vi "AO 1 Samples FPGA（Host）.vi"() -> ()   [LabVIEW 2019]
uses:
  <vilib>/FPGAPlugInAG/ELVIS III/niLvFpga_Open_ELVIS III.vi
  <vilib>/rvi/interface/common/dynamic/niFpgaDynamicAddResources.vi
  <vilib>/Utility/error.llb/Error Cluster From Error Code.vi
  <vilib>/rvi/errors/niLvFpgaAdjustHostInterfaceError.vi
  <vilib>/FPGAPlugInAG/Dynamic/niLvFpga_Run_Dynamic.vi
  <vilib>/FPGAPlugInAG/Dynamic/niLvFpga_Close_Dynamic.vi
  <vilib>/rvi/interface/nirviOpenFPGA/nirviOpenFPGA.xnode
  FPGA Bitfiles/analogio-fpga_FPGATarget_AO1SamplesFPGA_Fh4Y4n0B4rI.lvbitx
  AO 1 Samples FPGA.vi
  <vilib>/rvi/interface/nirviReadWriteControl/nirviReadWriteControl.xnode
  <vilib>/rvi/interface/nirviMethod/nirviMethod.xnode
  <vilib>/rvi/interface/nirviCloseFPGA/nirviCloseFPGA.xnode
  NiFpgaLv.dll
  <vilib>/rvi/interface/Simulation/niFpgaSimulationCallBeginRW.vi
panel:
  in  "停止":bool
  in  "B1":dbl
  in  "B0":dbl
  in  "A1":dbl
  in  "A0":dbl
  in  "Enable":bool[](array[boolean])=[TRUE, FALSE, FALSE, FALSE]
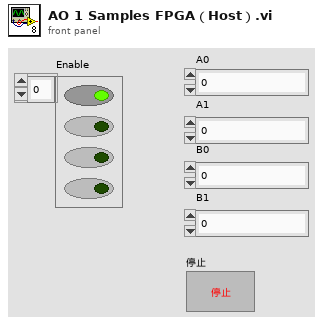
[diagram p1: front panel]
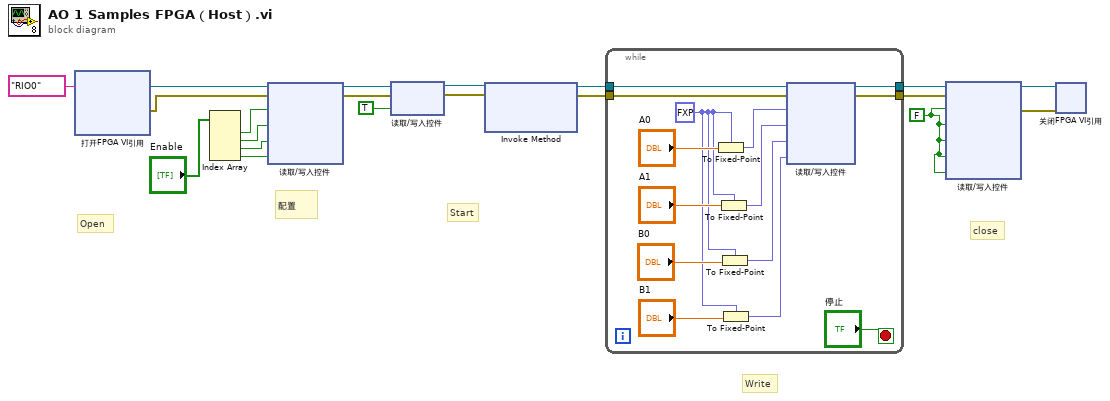
[diagram p0: block diagram]
diagram:
  w1 = FALSE
  # "Open"
  # "close"
  # "Write"
  # "Start"
  # "配置"
  n1 = xnode "打开FPGA VI引用"("资源名称"=tag "RIO0") -> ("FPGA VI引用输出"=w18:refnum<k20>, "错误输出"=w17:errorcluster)  [unwired: 1 in]
  n2 = Index Array(array="Enable") -> (element #1=w16:bool, element #2=w13:bool, element #3=w15:bool, element #4=w14:bool)  [unwired: 4 in]
  n3 = xnode "读取/写入控件"("FPGA VI引用输入"=w18, "错误输入"=w17, "A0.Enable"=w16, "A1.Enable"=w13, "B0.Enable"=w15, "B1.Enable"=w14) -> ("FPGA VI引用输出"=w11:refnum<k20>, "错误输出"=w12:errorcluster)
  n4 = xnode "读取/写入控件"("FPGA VI引用输入"=w11, "错误输入"=w12, "开始"=TRUE) -> ("FPGA VI引用输出"=w8:refnum<k20>, "错误输出"=w9:errorcluster)
  n5 = xnode "Invoke Method"("FPGA VI引用输入"=w8, "错误输入"=w9) -> ("FPGA VI引用输出"=w6:refnum<k20>, "错误输出"=w7:errorcluster)  [unwired: 1 in]
  n6 = while {
    tunnel: w7 -> [w34]
    tunnel: w6 -> [w33]
    tunnel: [w23] -> w5
    tunnel: [w22] -> w4
    stop <- "停止" stop-if-true
    w24 = fxp<+/-,20,5> 0.0 ("定点类型")
    n7 = To Fixed-Point(fixed-point type=w24, number="A0") -> (fixed-point=w31:fxp<+/-,20,5>)
    n8 = To Fixed-Point(fixed-point type=w24, number="A1") -> (fixed-point=w27:fxp<+/-,20,5>)
    n9 = To Fixed-Point(fixed-point type=w24, number="B0") -> (fixed-point=w25:fxp<+/-,20,5>)
    n10 = To Fixed-Point(fixed-point type=w24, number="B1") -> (fixed-point=w26:fxp<+/-,20,5>)
    n11 = xnode "读取/写入控件"("FPGA VI引用输入"=w33, "错误输入"=w34, "A0.Value"=w31, "A1.Value"=w27, "B0.Value"=w25, "B1.Value"=w26) -> ("FPGA VI引用输出"=w22:refnum<k20>, "错误输出"=w23:errorcluster)
  }
  n12 = xnode "读取/写入控件"("FPGA VI引用输入"=w4, "错误输入"=w5, "A0.Enable"=w1, "A1.Enable"=w1, "B0.Enable"=w1, "B1.Enable"=w1, "开始"=w1) -> ("FPGA VI引用输出"=w2:refnum<k20>, "错误输出"=w3:errorcluster)
  n13 = xnode "关闭FPGA VI引用"("FPGA VI引用输入"=w2, "错误输入"=w3) -> ()  [unwired: 1 out]
